vi "CS_MFA_LED_Status_D2-GREEN.vi"() -> ()   [LabVIEW 2018]
panel:
  out "error MotorTestMode 0":errorcluster
  out "error MotorTestMode 1":errorcluster
  out "error MotorTestMode 2":errorcluster
  out "error MotorTestMode 3":errorcluster
  out "AAABuild":i32
  in  "MintController":refnum<k7>(container)
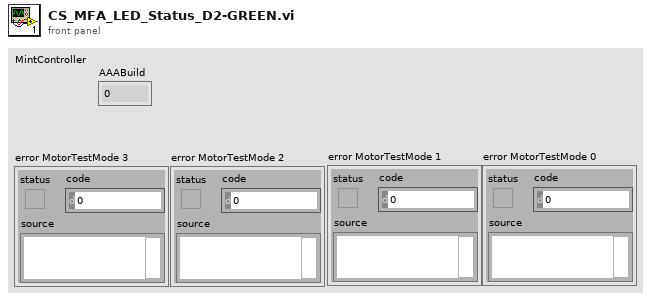
[diagram p1: front panel]
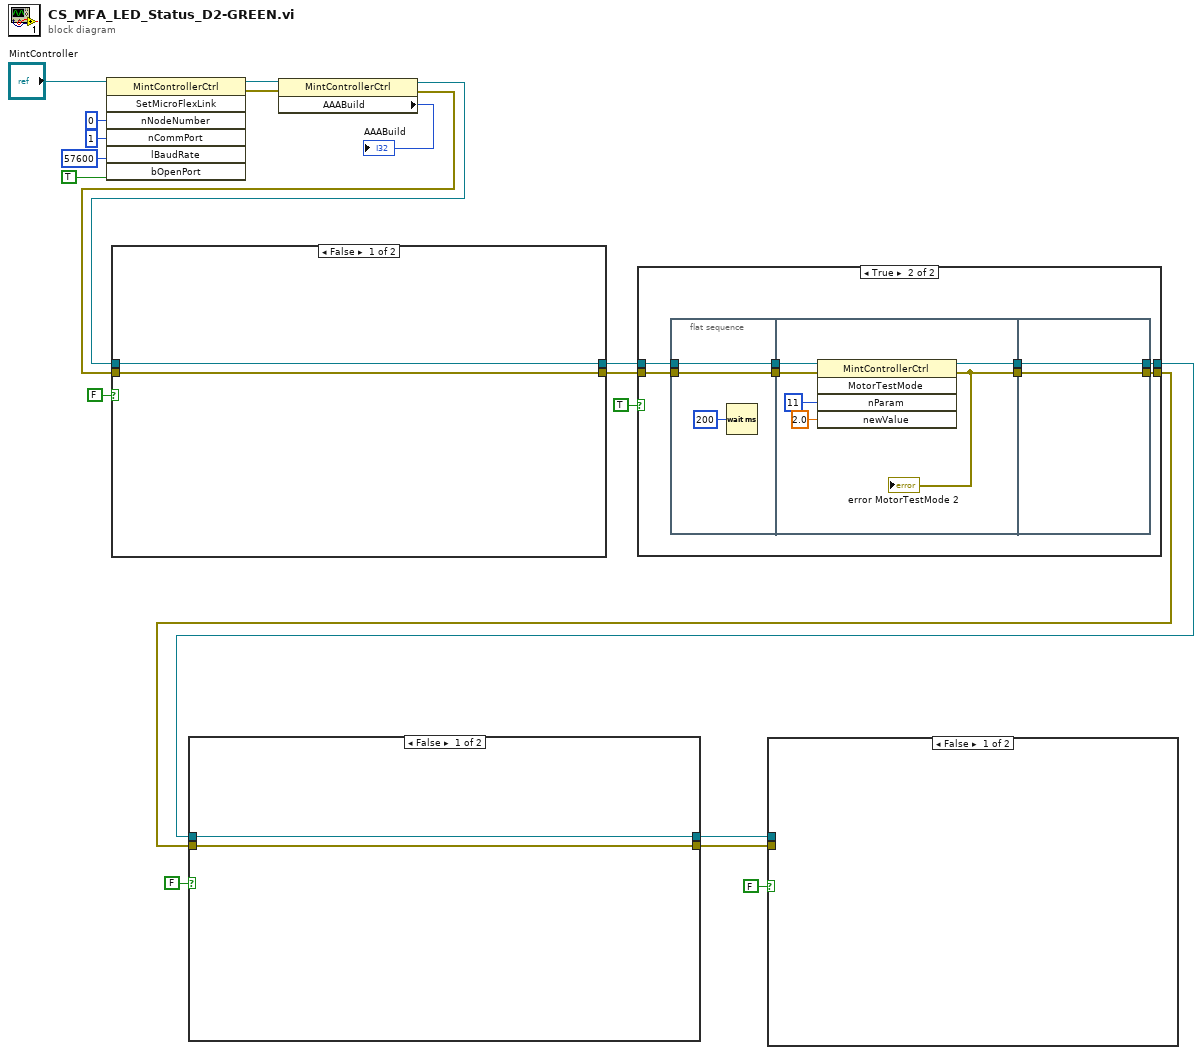
[diagram p0: block diagram]
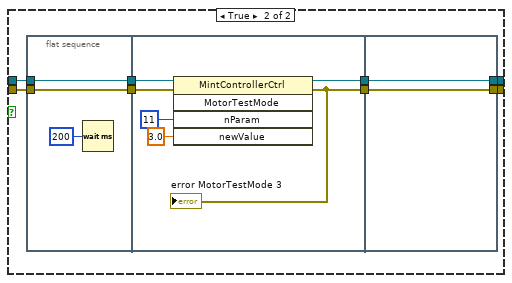
[diagram p2: hidden frame]
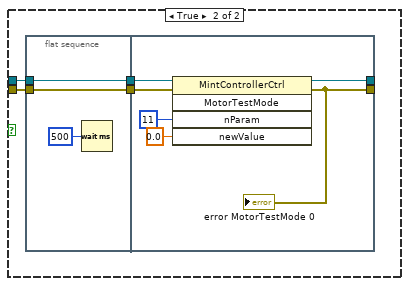
[diagram p3: hidden frame]
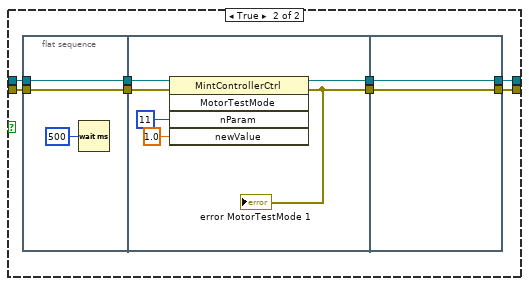
[diagram p4: hidden frame]
diagram:
  n1 = invoke class="MintControllerCtrl" method="SetMicroFlexLink"(reference="MintController", "nNodeNumber"=i16 0, "nCommPort"=i16 1, "lBaudRate"=57600, "bOpenPort"=TRUE) -> (reference out=w20:refnum<k7>, error out=w14:errorcluster)  [unwired: 2 in, 5 out]
  n2 = property class="MintControllerCtrl"(reference=w20, error in=w14) -> (reference out=w12:refnum<k7>, error out=w11:errorcluster, "AAABuild"=→"AAABuild":i32)
  n3 = case shown="False" FALSE {
    tunnel: w12 -> [w22 w26]
    tunnel: w11 -> [w21 w25]
    tunnel: [w22 w24] -> w10
    tunnel: [w21 w23] -> w9
    frame False {
    }
    frame True {
      n4 = flat-sequence {
        tunnel: [w31] -> w30
        tunnel: [w32] -> w29
        tunnel: w26 -> [w32]
        tunnel: w25 -> [w31]
        tunnel: w30 -> [w38]
        tunnel: w29 -> [w39]
        tunnel: [w35] -> w28
        tunnel: [w34] -> w27
        tunnel: [w40] -> w23
        tunnel: [w41] -> w24
        tunnel: w28 -> [w41]
        tunnel: w27 -> [w40]
        frame #0 {
          n5 = Wait (ms)(milliseconds to wait=u32 200) -> ()  [unwired: 1 out]
        }
        frame #1 {
          n6 = invoke class="MintControllerCtrl" method="MotorTestMode"(reference=w39, error in=w38, "nParam"=i16 11, "newValue"=sgl 3.0) -> (reference out=w35:refnum<k7>, error out=w34:errorcluster)  [unwired: 1 in, 3 out]
          "error MotorTestMode 3" <- w34
        }
        frame #2 {
        }
      }
    }
  }
  n7 = case shown="True" TRUE {
    tunnel: w10 -> [w43 w47]
    tunnel: w9 -> [w42 w46]
    tunnel: [w43 w45] -> w7
    tunnel: [w42 w44] -> w6
    frame False {
    }
    frame True {
      n8 = flat-sequence {
        tunnel: [w52] -> w51
        tunnel: [w53] -> w50
        tunnel: w47 -> [w53]
        tunnel: w46 -> [w52]
        tunnel: w51 -> [w59]
        tunnel: w50 -> [w60]
        tunnel: [w56] -> w49
        tunnel: [w55] -> w48
        tunnel: [w61] -> w44
        tunnel: [w62] -> w45
        tunnel: w49 -> [w62]
        tunnel: w48 -> [w61]
        frame #0 {
          n9 = Wait (ms)(milliseconds to wait=u32 200) -> ()  [unwired: 1 out]
        }
        frame #1 {
          n10 = invoke class="MintControllerCtrl" method="MotorTestMode"(reference=w60, error in=w59, "nParam"=i16 11, "newValue"=sgl 2.0) -> (reference out=w56:refnum<k7>, error out=w55:errorcluster)  [unwired: 1 in, 3 out]
          "error MotorTestMode 2" <- w55
        }
        frame #2 {
        }
      }
    }
  }
  n11 = case shown="False" FALSE {
    tunnel: [w63 w68] -> w8
    tunnel: w7 -> [w64 w67]
    tunnel: w6 -> [w63 w66]
    tunnel: [w64 w65] -> w5
    frame False {
    }
    frame True {
      n12 = flat-sequence {
        tunnel: [w73] -> w72
        tunnel: [w74] -> w71
        tunnel: w67 -> [w74]
        tunnel: w66 -> [w73]
        tunnel: w72 -> [w80]
        tunnel: w71 -> [w81]
        tunnel: [w77] -> w70
        tunnel: [w76] -> w69
        tunnel: [w82] -> w68
        tunnel: [w83] -> w65
        tunnel: w70 -> [w83]
        tunnel: w69 -> [w82]
        frame #0 {
          n13 = Wait (ms)(milliseconds to wait=u32 500) -> ()  [unwired: 1 out]
        }
        frame #1 {
          n14 = invoke class="MintControllerCtrl" method="MotorTestMode"(reference=w81, error in=w80, "nParam"=i16 11, "newValue"=sgl 1.0) -> (reference out=w77:refnum<k7>, error out=w76:errorcluster)  [unwired: 1 in, 3 out]
          "error MotorTestMode 1" <- w76
        }
        frame #2 {
        }
      }
    }
  }
  n15 = case shown="False" FALSE {
    tunnel: w8 -> [_ w85]
    tunnel: w5 -> [_ w84]
    frame False {
    }
    frame True {
      n16 = flat-sequence {
        tunnel: [w88] -> w87
        tunnel: [w89] -> w86
        tunnel: w84 -> [w89]
        tunnel: w85 -> [w88]
        tunnel: w87 -> [w95]
        tunnel: w86 -> [w96]
        tunnel: [w92] -> _
        tunnel: [w91] -> _
        frame #0 {
          n17 = Wait (ms)(milliseconds to wait=u32 500) -> ()  [unwired: 1 out]
        }
        frame #1 {
          n18 = invoke class="MintControllerCtrl" method="MotorTestMode"(reference=w96, error in=w95, "nParam"=i16 11, "newValue"=sgl 0.0) -> (reference out=w92:refnum<k7>, error out=w91:errorcluster)  [unwired: 1 in, 3 out]
          "error MotorTestMode 0" <- w91
        }
      }
    }
  }
